vi "Pause AE.vi"(1 "Pause In":bool, 2 "Action":T1) -> (0 "Pause Out":bool)   [LabVIEW 2014]
uses:
  Controls/Standard Action for Focus Lock.ctl
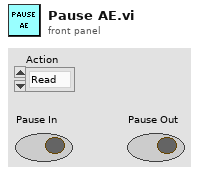
[diagram p1: front panel]
types:
  T1 = typedef "Standard Action for Focus Lock.ctl" = enum16{"Read", "Write"}
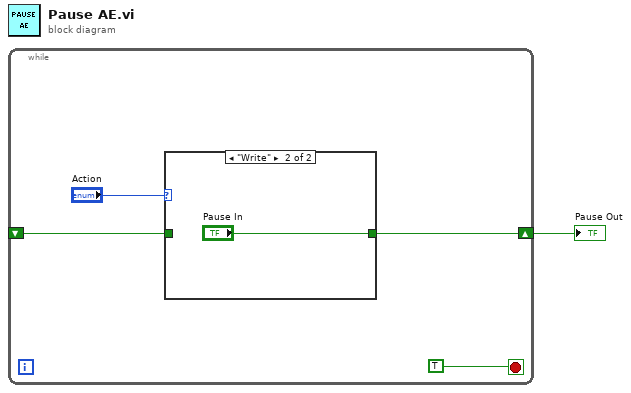
[diagram p0: block diagram]
diagram:
  n1 = while {
    shift-right: [w5] -> w1
    shift-left: _ -> [w4]
    stop <- TRUE stop-if-true
    n2 = case shown="\"Write\"" "Action" {
      tunnel: [w6 "Pause In"] -> w5
      tunnel: w4 -> [w6 _]
      frame "Read", Default {
      }
      frame "Write" {
      }
    }
  }
  "Pause Out" <- w1
